vi "数组插入函数.vi"() -> ()   [LabVIEW 2012]
panel:
  out "输出数组 4":i32[](array[numeric])
  out "输出数组 3":i32[](array[numeric])
  out "输出数组 2":i32[](array[numeric])
  out "输出数组":i32[](array[numeric])
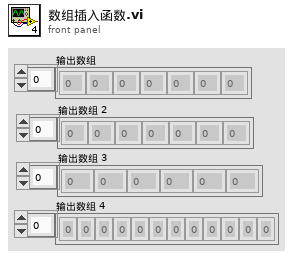
[diagram p1: front panel]
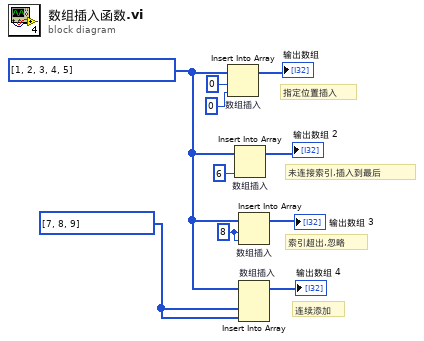
[diagram p0: block diagram]
diagram:
  w2 = i32[] [7, 8, 9]
  w5 = 8 ("索引")
  w3 = i32[] [1, 2, 3, 4, 5]
  # "指定位置插入"
  # "连续添加"
  # "索引超出,忽略"
  # "未连接索引,插入到最后"
  n1 = Insert Into Array "数组插入"(array=w3, index=0 ("索引"), new element=0 ("新元素/子数组")) -> (→"输出数组":i32[])
  n2 = Insert Into Array "数组插入"(array=w3, new element=6 ("新元素/子数组")) -> (→"输出数组 2":i32[])  [unwired: 1 in]
  n3 = Insert Into Array "数组插入"(array=w3, index=w5, new element=w5) -> (→"输出数组 3":i32[])
  n4 = Insert Into Array "数组插入"(array=w3, new element #1=w2, new element #2=w2) -> (→"输出数组 4":i32[])  [unwired: 1 in]
